vi "Apend Assertion Result.vi"(8 "error in (no error)":errorcluster, 9 "Assertion Result":T1, 11 "Plain Text Report In":refnum<class "Plain Text Report.lvclass">) -> (0 "error out":errorcluster, 3 "Plain Text Report Out":refnum<class "Plain Text Report.lvclass">)   [LabVIEW 2020, in "Plain Text Report.lvclass"]
uses:
  Plain Text Report.lvclass
  Result Types/Assertion Result/Assertion Result.ctl
  Result Types/Assertion Result/Public/TypeDefs/Status.ctl
  Result Types/Assertion Result/Public/TypeDefs/Assertion Type.ctl
  Result Types/Assertion Result/Assertion Result.lvlib
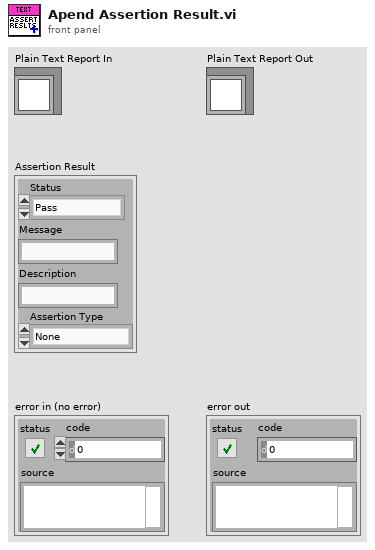
[diagram p1: front panel]
types:
  T1 = typedef "Assertion Result.lvlib/Assertion Result.ctl" = cluster{"Status":T2, "Message":string, "Description":string, "Assertion Type":T3}
  T2 = typedef "Assertion Result.lvlib/Status.ctl" = enum16{"Pass", "Fail", "Error", "Skipped", "Setup Error", "Broken", "Teardown Error"}
  T3 = typedef "Assertion Result.lvlib/Assertion Type.ctl" = enum16{"None", "Pass", "Fail", "Skip", "Pass if Equal", "Fail if Equal", "Pass if Error", "Fail if Error", "Pass if", "Fail if"}
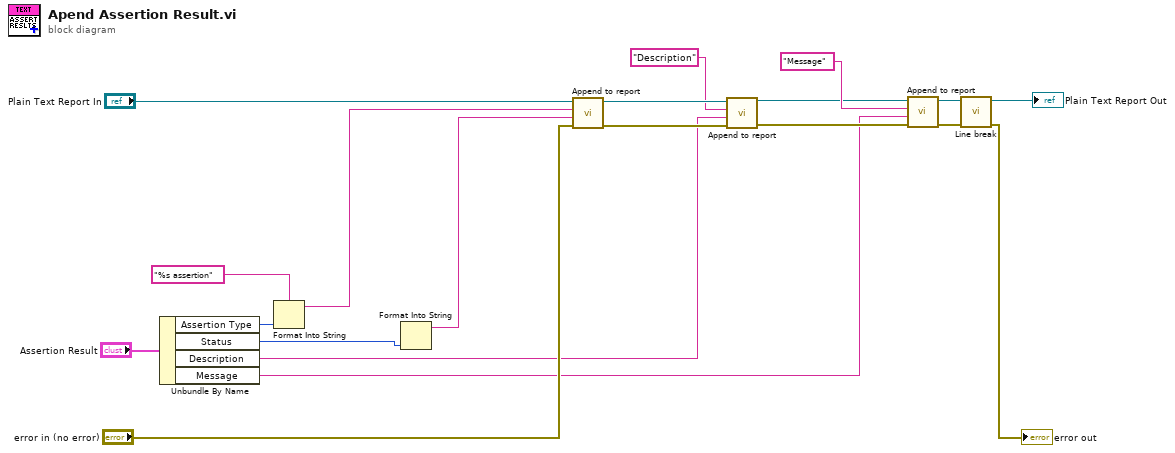
[diagram p0: block diagram]
diagram:
  n1 = Unbundle By Name("Assertion Result") -> ("Assertion Type"=w4:T3, "Status"=w1:T2, "Description"=w2:string, "Message"=w3:string)
  n2 = Format Into String(format string="%s assertion", w4) -> (resulting string=w18:string)  [unwired: 2 in, 1 out]
  n3 = Format Into String(w1) -> (resulting string=w17:string)  [unwired: 3 in, 1 out]
  n4 = call "Append to report.vi"("error in (no error)"="error in (no error)", "Value"=w17, "Key"=w18, "Plain Text Report In"="Plain Text Report In") -> ("error out"=w7:errorcluster, "Plain Text Report Out"=w16:refnum<class "Plain Text Report.lvclass">)  [unwired: 6 in]
  n5 = call "Append to report.vi"("error in (no error)"=w7, "Value"=w2, "Key"="Description", "Plain Text Report In"=w16) -> ("error out"=w8:errorcluster, "Plain Text Report Out"=w13:refnum<class "Plain Text Report.lvclass">)  [unwired: 6 in]
  n6 = call "Append to report.vi"("error in (no error)"=w8, "Value"=w3, "Key"="Message", "Plain Text Report In"=w13) -> ("error out"=w10:errorcluster, "Plain Text Report Out"=w12:refnum<class "Plain Text Report.lvclass">)  [unwired: 6 in]
  n7 = call "Line break.vi"("error in (no error)"=w10, "Plain Text Report In"=w12) -> ("error out"=→"error out":errorcluster, "Plain Text Report Out"=→"Plain Text Report Out":refnum<class "Plain Text Report.lvclass">)  [unwired: 8 in]
